vi "MKS670_RS232_meas_p.vi"(8 "error in":errorcluster, 11 "VISA in":refnum<visa-resource-name>) -> (0 "error out":errorcluster, 2 "pressure":dbl, 3 "VISA out":refnum<visa-resource-name>, 4 "status":bool)   [LabVIEW 2019]
uses:
  <vilib>/Instr/_visa.llb/VISA Flush IO Buffer Mask.ctl
panel:
  out "status string":string
  out "Read buffer":string
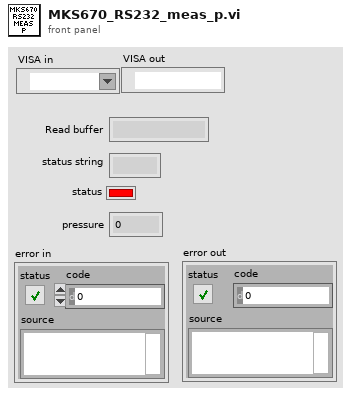
[diagram p1: front panel]
types:
  T1 = typedef "VISA Flush IO Buffer Mask.ctl" = u16
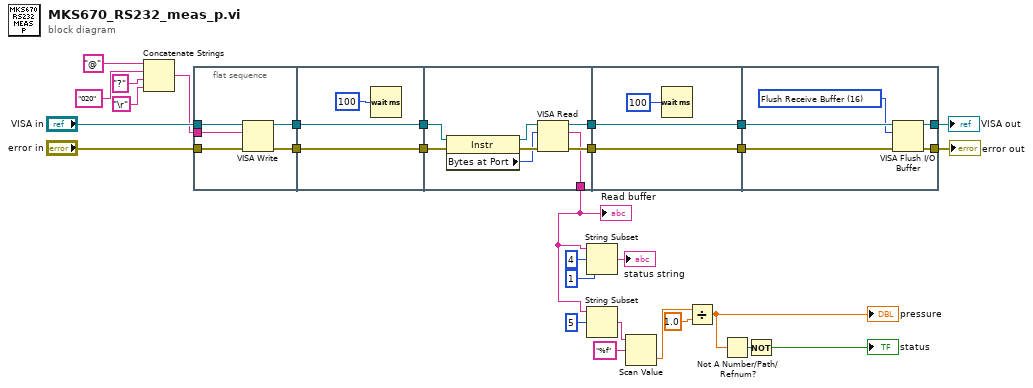
[diagram p0: block diagram]
diagram:
  n1 = Concatenate Strings("@" ("string"), "020" ("string"), "?" ("string"), "\r") -> (w12:string)
  n2 = flat-sequence {
    tunnel: w12 -> [w34]
    tunnel: "VISA in" -> [w33]
    tunnel: [w32] -> w29
    tunnel: [w31] -> w28
    tunnel: "error in" -> [w30]
    tunnel: w29 -> [w36]
    tunnel: [w36] -> w27
    tunnel: w28 -> [w35]
    tunnel: [w35] -> w26
    tunnel: w27 -> [w42]
    tunnel: w26 -> [w41]
    tunnel: [w40] -> w25
    tunnel: [w39] -> w24
    tunnel: [w38] -> w18
    tunnel: w25 -> [w48]
    tunnel: w24 -> [w47]
    tunnel: [w48] -> w23
    tunnel: [w47] -> w22
    tunnel: w23 -> [w53]
    tunnel: w22 -> [w52]
    tunnel: [w50] -> w3
    tunnel: [w49] -> w1
    frame #0 {
      n3 = VISA Write(VISA resource name=w33, write buffer=w34, error in (no error)=w30) -> (VISA resource name out=w32:refnum<visa-resource-name>, error out=w31:errorcluster)  [unwired: 1 out]
    }
    frame #1 {
      n4 = Wait (ms)(milliseconds to wait=u32 100) -> ()  [unwired: 1 out]
    }
    frame #2 {
      n5 = property class="Instr"(reference=w42, error in=w41) -> (reference out=w43:refnum<visa-resource-name>, error out=w45:errorcluster, "Bytes at Port"=w44:u32)
      n6 = VISA Read(VISA resource name=w43, byte count=w44, error in (no error)=w45) -> (VISA resource name out=w40:refnum<visa-resource-name>, read buffer=w38:string, error out=w39:errorcluster)  [unwired: 1 out]
    }
    frame #3 {
      n7 = Wait (ms)(milliseconds to wait=u32 100) -> ()  [unwired: 1 out]
    }
    frame #4 {
      w51 = T1 16 items=["Flush Receive Buffer"=16, "Write Transmit Buffer to Device"=32, "Flush Receive Buffer (No I/O)"=64, "Flush Transmit Buffer"=128] ("Mask")
      n8 = VISA Flush I/O Buffer(VISA resource name=w53, mask (16)=w51, error in (no error)=w52) -> (VISA resource name out=w50:refnum<visa-resource-name>, error out=w49:errorcluster)
    }
  }
  n9 = String Subset(string=w18, offset (0)=4, length (rest)=1 ("length (rest)")) -> (substring=→"status string":string)
  n10 = String Subset(string=w18, offset (0)=5) -> (substring=w19:string)  [unwired: 1 in]
  n11 = Scan Value(string=w19, format string="%f") -> (value=w21:dbl)  [unwired: 1 in, 1 out]
  n12 = Divide(x=w21, y=1.0) -> (x/y=w11:dbl)
  "pressure" <- w11
  n13 = Not A Number/Path/Refnum?(number/path/refnum=w11) -> (NaN/Path/Refnum?=w7:bool)
  n14 = Not(x=w7) -> (.not. x?=→"status":bool)
  "Read buffer" <- w18
  "VISA out" <- w3
  "error out" <- w1
